vi "color image 3d.vi"(5 "Z Slice":i16=2, 6 "path to JPEG file":path=path "E:/Dati/XRF/20200416 - faggio/tables 3d/figs", 7 "Max":i32=495, 8 "Names":T2={"Red name"="Sr", "Green name"="Cl", "Blu name"="Mn"}, 9 "ROI-Blue":i32[][](graph)=array9x561[5049 elements], 10 "ROI-Green":i32[][](graph)=array9x561[5049 elements], 11 "ROI-Red":i32[][](graph)=array9x561[5049 elements]) -> ()   [LabVIEW 2023]
uses:
  <vilib>/Utility/miscctls.llb/LVBoundsTypeDef.ctl
  <vilib>/vision/Management.llb/Cast Image 2 Method.ctl
  <vilib>/vision/NI_Vision_Development_Module.lvlib
panel:
  out "Blue":T1(plugin-control)
  out "Green":T1(plugin-control)
  out "Red":T1(plugin-control)
  out "concatenated string":picture
  out "error out":errorcluster
  in  "error in":errorcluster
  out "Intensity Graph 6":u16[][](graph)
  out "Intensity Graph 5":u16[][](graph)
  out "Intensity Graph 4":u16[][](graph)
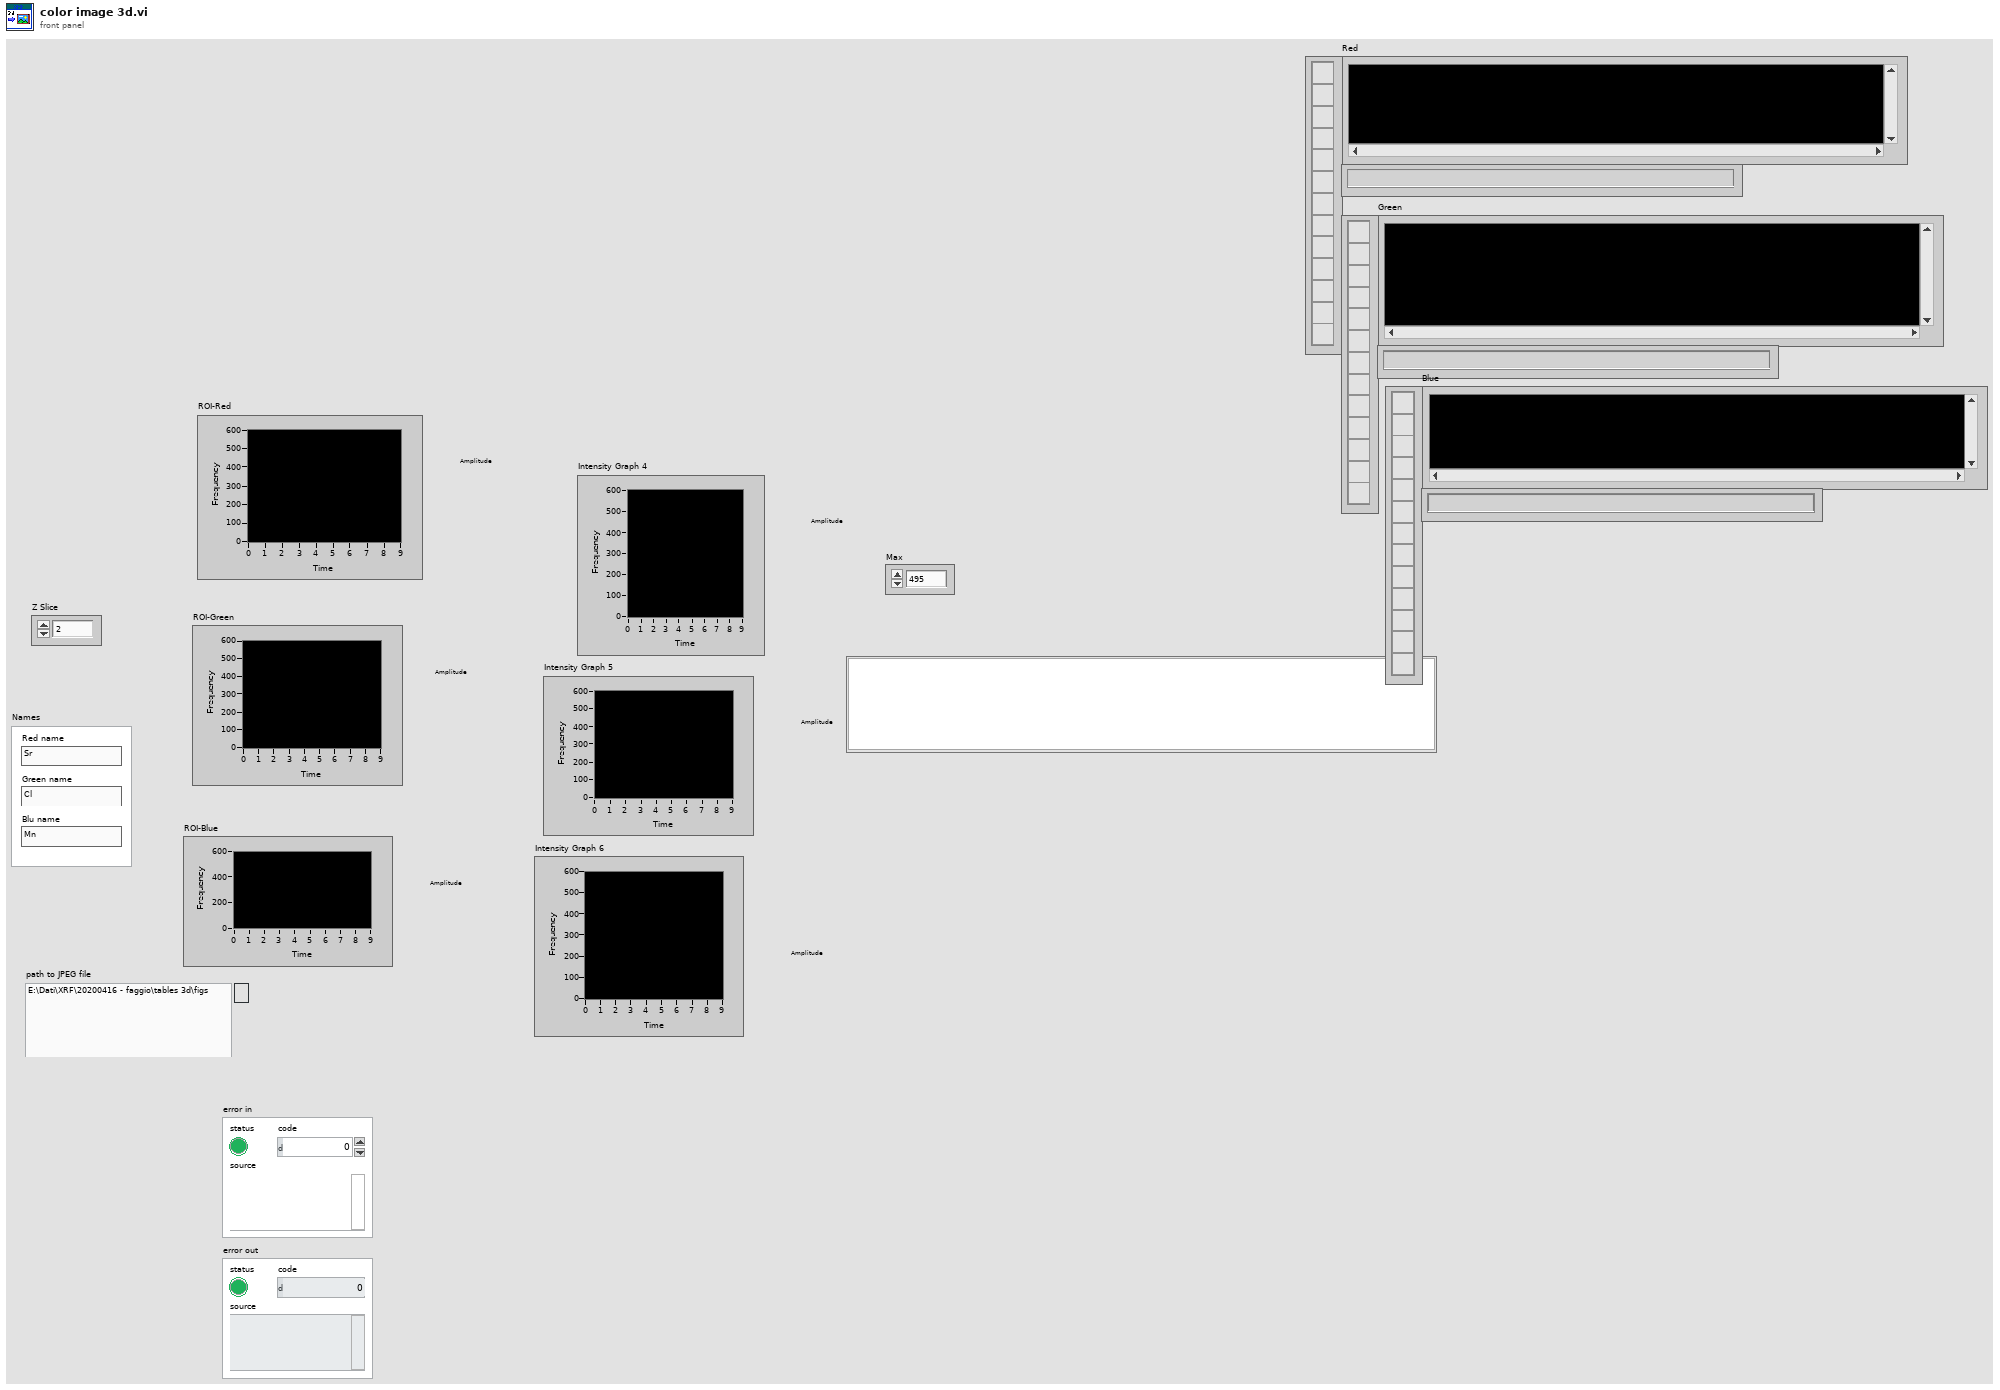
[diagram p1: front panel]
types:
  T1 = typedef "IMAQ Image.ctl" = refnum<image>
  T2 = cluster{"Red name":string, "Green name":string, "Blu name":string}
  T3 = typedef "Cast Image 2 Method.ctl" = u32
  T4 = typedef "Image Type" = u32
  T5 = typedef "LVBoundsTypeDef.ctl" = cluster{"Width":u32, "Height":u32}
  T6 = enum16{"User-specified Font", "Application Font", "System Font", "Dialog Font"}
  T7 = cluster{"Font Name:":string, "Size":i16, "Strikeout?":bool, "Italic?":bool, "Underline?":bool, "Outline?":bool, "Shadow?":bool, "Bold?":bool}
  T8 = typedef "imagedata.ctl" = cluster{"image type":i32, "image depth":i32, "image":u8[], "mask":u8[], "colors":u32[], "Rectangle":cluster{"left":i16, "top":i16, "right":i16, "bottom":i16}}
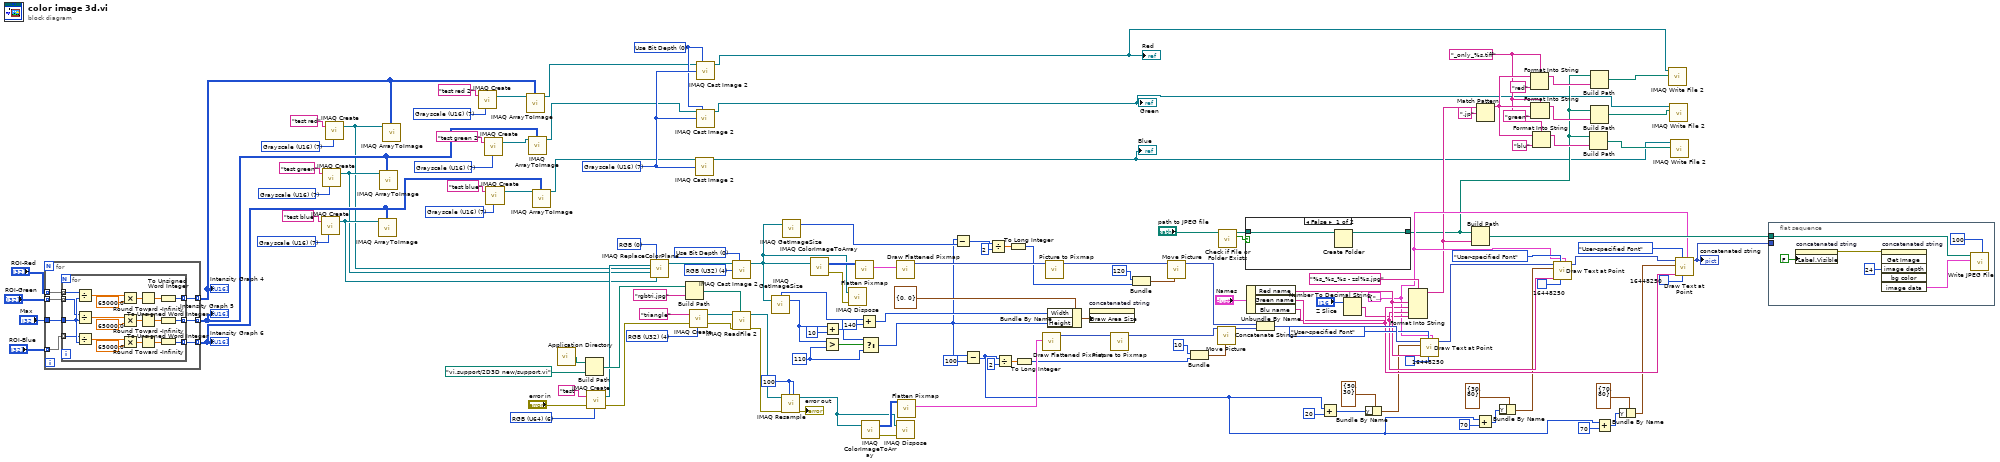
[diagram p0: block diagram]
diagram:
  w7 = T3 0 items=["Use Bit Depth", "Shift", "Use Lookup Table"] ("Method")
  w8 = T4 7 items=["Grayscale (U8)", "Grayscale (I16)", "Grayscale (SGL)", "Complex (CSG)", "RGB (U32)", "HSL (U32)", "RGB (U64)", "Grayscale (U16)"] ("Image Type")
  w24 = "_only_%s.tiff" ("format string")
  w58 = u32 110 ("Height")
  w61 = u16 0 items=["RGB", "HSL", "HSV", "HSI"] ("Color Mode")
  w75 = T4 7 items=["Grayscale (U8)", "Grayscale (I16)", "Grayscale (SGL)", "Complex (CSG)", "RGB (U32)", "HSL (U32)", "RGB (U64)", "Grayscale (U16)"] ("Image Type")
  w73 = T4 7 items=["Grayscale (U8)", "Grayscale (I16)", "Grayscale (SGL)", "Complex (CSG)", "RGB (U32)", "HSL (U32)", "RGB (U64)", "Grayscale (U16)"] ("Image Type")
  w72 = T4 7 items=["Grayscale (U8)", "Grayscale (I16)", "Grayscale (SGL)", "Complex (CSG)", "RGB (U32)", "HSL (U32)", "RGB (U64)", "Grayscale (U16)"] ("Image Type")
  w65 = T4 7 items=["Grayscale (U8)", "Grayscale (I16)", "Grayscale (SGL)", "Complex (CSG)", "RGB (U32)", "HSL (U32)", "RGB (U64)", "Grayscale (U16)"] ("Image Type")
  w68 = T4 7 items=["Grayscale (U8)", "Grayscale (I16)", "Grayscale (SGL)", "Complex (CSG)", "RGB (U32)", "HSL (U32)", "RGB (U64)", "Grayscale (U16)"] ("Image Type")
  w69 = T4 7 items=["Grayscale (U8)", "Grayscale (I16)", "Grayscale (SGL)", "Complex (CSG)", "RGB (U32)", "HSL (U32)", "RGB (U64)", "Grayscale (U16)"] ("Image Type")
  w85 = T4 4 items=["Grayscale (U8)", "Grayscale (I16)", "Grayscale (SGL)", "Complex (CSG)", "RGB (U32)", "HSL (U32)", "RGB (U64)", "Grayscale (U16)"] ("Image Type")
  w86 = T3 0 items=["Use Bit Depth", "Shift", "Use Lookup Table"] ("Method")
  w14 = T7 {"Font Name:"="Times", "Size"=18, "Strikeout?"=FALSE, "Italic?"=FALSE, "Underline?"=FALSE, "Outline?"=FALSE, "Shadow?"=FALSE, "Bold?"=TRUE} ("[user-specified font]")
  w124 = T4 4 items=["Grayscale (U8)", "Grayscale (I16)", "Grayscale (SGL)", "Complex (CSG)", "RGB (U32)", "HSL (U32)", "RGB (U64)", "Grayscale (U16)"] ("Image Type")
  w128 = 100
  w137 = T4 6 items=["Grayscale (U8)", "Grayscale (I16)", "Grayscale (SGL)", "Complex (CSG)", "RGB (U32)", "HSL (U32)", "RGB (U64)", "Grayscale (U16)"] ("Image Type")
  n1 = for {
    tunnel: "ROI-Red" -> [w149] mode=indexing
    tunnel: "ROI-Green" -> [w148] mode=indexing
    tunnel: "ROI-Blue" -> [w147] mode=indexing
    tunnel: "Max" -> [w146]
    tunnel: [w145] -> w64 mode=indexing
    tunnel: [w144] -> w63 mode=indexing
    tunnel: [w143] -> w62 mode=indexing
    n2 = for {
      tunnel: w149 -> [w168] mode=indexing
      tunnel: w148 -> [w158] mode=indexing
      tunnel: w147 -> [w159] mode=indexing
      tunnel: w146 -> [w160]
      tunnel: [w165] -> w145 mode=indexing
      tunnel: [w157] -> w144 mode=indexing
      tunnel: [w156] -> w143 mode=indexing
      n3 = Divide(x=w168, y=w160) -> (x/y=w153:dbl)
      n4 = Divide(x=w158, y=w160) -> (x/y=w154:dbl)
      n5 = Divide(x=w159, y=w160) -> (x/y=w155:dbl)
      n6 = Multiply(x=w153, y=65000.0) -> (x*y=w166:dbl)
      n7 = Multiply(x=w154, y=65000.0) -> (x*y=w164:dbl)
      n8 = Multiply(x=w155, y=65000.0) -> (x*y=w161:dbl)
      n9 = Round Toward -Infinity(1:w166) -> (0:w152:dbl)
      n10 = Round Toward -Infinity(1:w164) -> (0:w151:dbl)
      n11 = Round Toward -Infinity(1:w161) -> (0:w150:dbl)
      n12 = To Unsigned Word Integer(number=w152) -> (unsigned 16bit integer=w165:u16)
      n13 = To Unsigned Word Integer(number=w151) -> (unsigned 16bit integer=w157:u16)
      n14 = To Unsigned Word Integer(number=w150) -> (unsigned 16bit integer=w156:u16)
    }
  }
  "Intensity Graph 5" <- w63
  "Intensity Graph 6" <- w62
  "Intensity Graph 4" <- w64
  n15 = call "IMAQ Create"("Image Name"="test blue", "Image Type"=w65) -> ("New Image"=w11:T1)  [unwired: 3 in, 1 out]
  n16 = call "IMAQ Create"("Image Name"="test green", "Image Type"=w68) -> ("New Image"=w10:T1)  [unwired: 3 in, 1 out]
  n17 = call "IMAQ Create"("Image Name"="test red", "Image Type"=w69) -> ("New Image"=w9:T1)  [unwired: 3 in, 1 out]
  n18 = call "IMAQ ArrayToImage"("Image Pixels (U16)"=w62, "Image"=w11) -> ()  [unwired: 8 in, 2 out]
  n19 = call "IMAQ ArrayToImage"("Image Pixels (U16)"=w63, "Image"=w10) -> ()  [unwired: 8 in, 2 out]
  n20 = call "IMAQ ArrayToImage"("Image Pixels (U16)"=w64, "Image"=w9) -> ()  [unwired: 8 in, 2 out]
  n21 = call "IMAQ Create"("Image Name"="test red 2", "Image Type"=w72) -> ("New Image"=w78:T1)  [unwired: 3 in, 1 out]
  n22 = call "IMAQ Create"("Image Name"="test green 2", "Image Type"=w73) -> ("New Image"=w79:T1)  [unwired: 3 in, 1 out]
  n23 = call "IMAQ Create"("Image Name"="test blue", "Image Type"=w75) -> ("New Image"=w77:T1)  [unwired: 3 in, 1 out]
  n24 = call "IMAQ ArrayToImage"("Image Pixels (U16)"=w64, "Image"=w78) -> ("Image Out"=w1:T1)  [unwired: 8 in, 1 out]
  n25 = call "IMAQ ArrayToImage"("Image Pixels (U16)"=w63, "Image"=w79) -> ("Image Out"=w4:T1)  [unwired: 8 in, 1 out]
  n26 = call "IMAQ ArrayToImage"("Image Pixels (U16)"=w62, "Image"=w77) -> ("Image Out"=w6:T1)  [unwired: 8 in, 1 out]
  n27 = call <vilib>:"Application Directory.vi"() -> ("Application Directory"=w130:path)
  n28 = Build Path(base path=w130, name or relative path=path "vi.support/2D3D new/support.vi") -> (appended path=w131:path)
  n29 = call "IMAQ Create"("Image Name"="test", "Image Type"=w137, "error in (no error)"="error in") -> ("New Image"=w59:T1, "error out"=w99:errorcluster)  [unwired: 2 in]
  n30 = call "IMAQ ReplaceColorPlane"("Color Mode"=w61, "Image Dst"=w59, "Red or Hue Plane"=w9, "Green or Sat Plane"=w10, "Blue or Luma or Val or Inten Plane"=w11) -> ("Image Dst Out"=w60:T1)  [unwired: 9 in, 1 out]
  n31 = Build Path(base path=w131, name or relative path="rgbtri.jpg") -> (appended path=w132:path)
  n32 = call "IMAQ Create"("Image Name"="triangle", "Image Type"=w124, "error in (no error)"=w99) -> ("New Image"=w135:T1, "error out"=w134:errorcluster)  [unwired: 2 in]
  n33 = call "IMAQ Cast Image 2"("Image Src"=w6, "Image Type"=w8) -> ("Image Dst Out"=w5:T1)  [unwired: 12 in, 1 out]
  "Blue" <- w5
  n34 = call "IMAQ Cast Image 2"("Image Src"=w4, "Method"=w7, "Image Type"=w8) -> ("Image Dst Out"=w3:T1)  [unwired: 11 in, 1 out]
  "Green" <- w3
  n35 = call "IMAQ Cast Image 2"("Image Src"=w1, "Method"=w7, "Image Type"=w8) -> ("Image Dst Out"=w2:T1)  [unwired: 11 in, 1 out]
  "Red" <- w2
  n36 = call "IMAQ Cast Image 2"("Image Src"=w60, "Method"=w86, "Image Type"=w85) -> ("Image Dst Out"=w46:T1)  [unwired: 11 in, 1 out]
  n37 = call "IMAQ ReadFile 2"("File Path"=w132, "error in (no error)"=w134, "Image"=w135) -> ("error out"=w125:errorcluster, "Image Out"=w127:T1)  [unwired: 4 in, 3 out]
  n38 = call "IMAQ GetImageSize"("Image"=w46) -> ("Y Resolution"=w51:i32, "X Resolution"=w52:i32)  [unwired: 3 in, 1 out]
  n39 = call "IMAQ Resample"("X Resolution"=w128, "Y Resolution"=w128, "error in (no error)"=w125, "Image Src"=w127) -> ("error out"=→"error out":errorcluster, "Image Dst Out"=w82:T1)  [unwired: 6 in]
  n40 = call "IMAQ GetImageSize"("Image"=w46) -> ("Y Resolution"=w47:i32)  [unwired: 3 in, 2 out]
  n41 = call "IMAQ ColorImageToArray"("Image"=w46) -> ("Image Pixels (U32)"=w123:u32[][], "error out"=w84:errorcluster)  [unwired: 3 in, 1 out]
  n42 = Greater?(x=w51, y=w58) -> (0:w55:bool)
  n43 = Add(x=w51, y=10) -> (x+y=w57:i32)
  n44 = call "IMAQ Dispose"("Image"=w46, "error in (no error)"=w84) -> ()  [unwired: 4 in, 1 out]
  n45 = call <vilib>:"Flatten Pixmap.vi"("24-bit pixmap"=w123) -> ("image data"=w122:T8)  [unwired: 10 in]
  n46 = Add(x=w52, y=140) -> (x+y=w53:i32)
  n47 = call "IMAQ ColorImageToArray"("Image"=w82) -> ("Image Pixels (U32)"=w120:u32[][], "error out"=w83:errorcluster)  [unwired: 3 in, 1 out]
  n48 = Select(t=w57, s=w55, f=w58) -> (s? t:f=w40:u32)
  n49 = call <vilib>:"Draw Flattened Pixmap.vi"("image data"=w122) -> ("new picture"=w119:picture)  [unwired: 8 in]
  n50 = call "IMAQ Dispose"("Image"=w82, "error in (no error)"=w83) -> ()  [unwired: 4 in, 1 out]
  n51 = call <vilib>:"Flatten Pixmap.vi"("24-bit pixmap"=w120) -> ("image data"=w121:T8)  [unwired: 10 in]
  n52 = Subtract(x=w40, y=w47) -> (x-y=w50:u32)
  n53 = Subtract(x=w40, y=u32 100) -> (x-y=w30:u32)
  n54 = Divide(x=w50, y=2) -> (x/y=w49:dbl)
  n55 = Divide(x=w30, y=2) -> (x/y=w42:dbl)
  n56 = To Long Integer(number=w49) -> (32bit integer=w45:i32)
  n57 = To Long Integer(number=w42) -> (32bit integer=w41:i32)
  n58 = call <vilib>:"Draw Flattened Pixmap.vi"("image data"=w121) -> ("new picture"=w118:picture)  [unwired: 8 in]
  n59 = call <vilib>:"Picture to Pixmap.vi"("picture"=w119) -> ("new picture"=w114:picture)  [unwired: 9 in, 1 out]
  n60 = Bundle By Name(cluster=T5 {"Width"=0, "Height"=0} ("Draw Area Size"), "Width"=w53, "Height"=w40) -> (w97:T5)
  n61 = property on="concatenated string" class="Pict"("Draw Area Size"=w97) -> ()  [unwired: 2 in, 2 out]
  n62 = call <vilib>:"Picture to Pixmap.vi"("picture"=w118) -> ("new picture"=w117:picture)  [unwired: 9 in, 1 out]
  n63 = Bundle(120, w45) -> (w113:cluster{i32, i32})  [unwired: 1 in]
  n64 = call "Move Picture.vi"("Delta"=w113, "Picture In"=w114) -> ("value"=w111:picture)  [unwired: 8 in, 1 out]
  n65 = Bundle(10, w41) -> (w116:cluster{i32, i32})  [unwired: 1 in]
  n66 = call "Move Picture.vi"("Delta"=w116, "Picture In"=w117) -> ("value"=w115:picture)  [unwired: 8 in, 1 out]
  n67 = call <vilib>:"Check if File or Folder Exists.vi"("path"="path to JPEG file") -> ("file or folder exists?"=w94:bool, "dup path"=w93:path)  [unwired: 8 in, 1 out]
  n68 = case shown="False" w94 {
    tunnel: [w169 w171] -> w12
    tunnel: w93 -> [w170 w171]
    frame False {
      n69 = Create Folder(path (use dialog)=w170) -> (created path=w169:path)  [unwired: 2 in, 2 out]
    }
    frame True {
    }
  }
  n70 = Unbundle By Name("Names") -> ("Red name"=w91:string, "Green name"=w90:string, "Blu name"=w89:string)
  n71 = Concatenate Strings(w111, w115) -> (w109:picture)
  n72 = Add(x=w30, y=u32 20) -> (x+y=w37:u32)
  n73 = Number To Decimal String(number="Z Slice") -> (decimal integer string=w81:string)  [unwired: 1 in]
  n74 = Bundle By Name(cluster=cluster{"x":i16, "y":i16} {"x"=50, "y"=30} ("origin"), "y"=w37) -> (w29:cluster{"x":i16, "y":i16})
  n75 = Format Into String(format string="%s_%s_%s - zsl%s.jpg", w91, w90, w89, w81) -> (resulting string=w13:string)  [unwired: 2 in, 1 out]
  n76 = call <vilib>:"Draw Text at Point.vi"("[user-specified font]"=w14, "text color(black)"=u32 16448250, "desired font(Application)"=T6."User-specified Font", "text"=w91, "origin"=w29, "picture"=w109) -> ("new picture"=w102:picture)  [unwired: 4 in, 1 out]
  n77 = Build Path(base path=w12, name or relative path=w13) -> (appended path=w88:path)
  n78 = Add(x=w30, y=u32 70) -> (x+y=w34:u32)
  n79 = Match Pattern(string=w13, regular expression=".jp") -> (before substring=w25:string)  [unwired: 1 in, 3 out]
  n80 = Bundle By Name(cluster=cluster{"X":i32, "Y":i32} {"X"=30, "Y"=80} ("Origin"), "Y"=w34) -> (w28:cluster{"X":i32, "Y":i32})
  n81 = Format Into String(format string=w24, initial string=w25, "red" ("input 1")) -> (resulting string=w20:string)  [unwired: 1 in, 1 out]
  n82 = Format Into String(format string=w24, initial string=w25, "green" ("input 1")) -> (resulting string=w19:string)  [unwired: 1 in, 1 out]
  n83 = Format Into String(format string=w24, initial string=w25, "blu" ("input 1")) -> (resulting string=w18:string)  [unwired: 1 in, 1 out]
  n84 = call <vilib>:"Draw Text at Point.vi"("[user-specified font]"=w14, "text color(black)"=u32 16448250, "desired font(Application)"=T6."User-specified Font", "text"=w89, "origin"=w28, "picture"=w102) -> ("new picture"=w101:picture)  [unwired: 4 in, 1 out]
  n85 = Build Path(base path=w12, name or relative path=w18) -> (appended path=w15:path)
  n86 = Build Path(base path=w12, name or relative path=w20) -> (appended path=w17:path)
  n87 = Build Path(base path=w12, name or relative path=w19) -> (appended path=w16:path)
  n88 = Add(x=w30, y=u32 70) -> (x+y=w33:u32)
  n89 = Bundle By Name(cluster=cluster{"X":i32, "Y":i32} {"X"=70, "Y"=80} ("Origin"), "Y"=w33) -> (w27:cluster{"X":i32, "Y":i32})
  n90 = call-poly "IMAQ Write File 2"("File Path"=w17, "Image"=w2) -> ()  [unwired: 8 in, 2 out]
  n91 = call-poly "IMAQ Write File 2"("File Path"=w16, "Image"=w3) -> ()  [unwired: 8 in, 2 out]
  n92 = call-poly "IMAQ Write File 2"("File Path"=w15, "Image"=w5) -> ()  [unwired: 8 in, 2 out]
  n93 = call <vilib>:"Draw Text at Point.vi"("[user-specified font]"=w14, "text color(black)"=u32 16448250, "desired font(Application)"=T6."User-specified Font", "text"=w90, "origin"=w27, "picture"=w101) -> ("new picture"=w87:picture)  [unwired: 4 in, 1 out]
  "concatenated string" <- w87
  n94 = flat-sequence {
    tunnel: w87 -> [_]
    tunnel: w88 -> [w176]
    frame #0 {
      n95 = property on="concatenated string" class="Pict"("Label.Visible"=FALSE) -> (error out=w174:errorcluster)  [unwired: 2 in, 1 out]
      n96 = invoke on="concatenated string" class="Pict" method="Get Image"(error in=w174, "image depth"=24 ("Image Depth")) -> ("image data"=w177:T8)  [unwired: 4 in, 5 out]
      n97 = call <vilib>:"Write JPEG File.vi"("quality (80)"=100, "image data"=w177, "path to JPEG file"=w176) -> ()  [unwired: 7 in, 2 out]
    }
  }
